vi "Help Ctrl Ref.vi"(9 "Operation":enum16{"Get", "Set"}(ring), 11 "Bool Refnum":refnum<vi>) -> (3 "Ctl Refnum (out)":refnum<vi>)   [LabVIEW 2017, in "WebServiceImporter.lvlib" / "Main Panel.lvlib"]
uses:
  <vilib>/Platform/WebService/Main Panel/Main Panel.lvlib
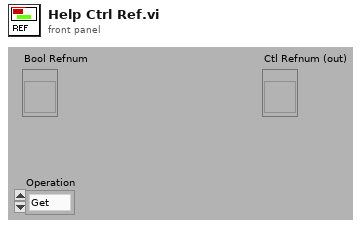
[diagram p1: front panel]
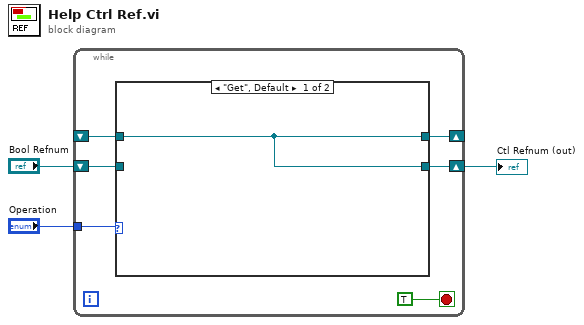
[diagram p0: block diagram]
diagram:
  n1 = while {
    tunnel: "Operation" -> [w8]
    shift-right: [w6] -> w1
    shift-left: "Bool Refnum" -> [w7]
    shift-right: [w5] -> _
    shift-left: _ -> [w4]
    stop <- TRUE stop-if-true
    n2 = case shown="\"Get\", Default" w8 {
      tunnel: w7 -> [_ w11]
      tunnel: [w10 w11] -> w6
      tunnel: [w10 w11] -> w5
      tunnel: w4 -> [w10 _]
      frame "Get", Default {
      }
      frame "Set" {
      }
    }
  }
  "Ctl Refnum (out)" <- w1
